vi "Preview Steps.vi"(11 "Actor in":refnum<class "Actor.lvclass">) -> (3 "Actor out":refnum<class "Actor.lvclass">, 5 "Steps":T1[](array[typedef]), 7 "Number Of Steps":i32)   [LabVIEW 2015, in "Actor.lvclass"]
uses:
  Actor.lvclass
  Sequencer/Single Step Data.ctl
  Messaging/Message/Message.lvclass
  Actor.lvclass/Actor.ctl
  Sequencer/Sequencer.lvclass/Sequencer.ctl
  Sequencer/Sequencer.lvclass
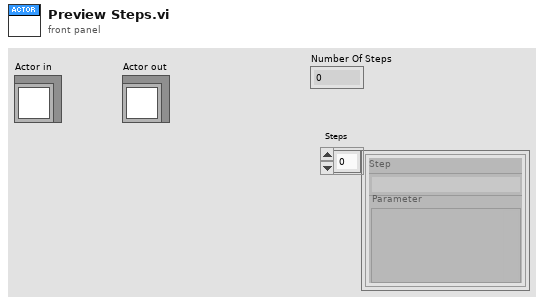
[diagram p1: front panel]
types:
  T1 = typedef "Sequencer.lvclass/Single Step Data.ctl" = cluster{"Step":string, "Parameter":variant, "Reply Channel":refnum<notifier>}
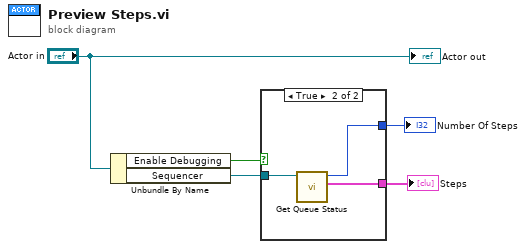
[diagram p0: block diagram]
diagram:
  n1 = Unbundle By Name("Actor in") -> ("Enable Debugging"=w2:bool, "Sequencer"=w5:refnum<class "Sequencer.lvclass">)
  n2 = case shown="True" w2 {
    tunnel: w5 -> [_ w8]
    tunnel: [_ w7] -> w4
    tunnel: [_ w6] -> w3
    frame False {
    }
    frame True {
      n3 = call "Get Queue Status.vi"("Sequencer in"=w8) -> ("Steps"=w6:T1[], "Number Of Steps"=w7:i32)  [unwired: 9 in]
    }
  }
  "Number Of Steps" <- w4
  "Steps" <- w3
  "Actor out" <- "Actor in"
